vi "Set Speed.vi"(8 "error in (no error)":errorcluster, 10 "speed":dbl, 11 "Masterflex Settings in":T1={"VISA resource name"="", "Simulated?"=FALSE, "Pump Number"=1.0, "Reverse?"=FALSE} {"Pump Number" min=1.0 max=20.0 step=1.0}) -> (0 "error out":errorcluster, 1 "Connection Error":bool, 3 "Masterflex Settings out":T1={"VISA resource name"="", "Simulated?"=FALSE, "Pump Number"=1.0, "Reverse?"=FALSE} {"Pump Number" min=1.0 max=20.0 step=1.0})   [LabVIEW 2018, in "Masterflex 7550-30.lvlib"]
uses:
  Masterflex 7550-30.lvlib
  Controls/Settings Cluster.ctl
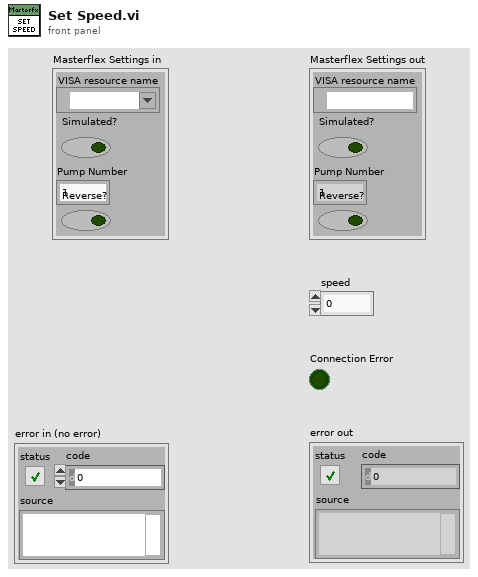
[diagram p1: front panel]
types:
  T1 = typedef "Masterflex 7550-30.lvlib/Settings Cluster.ctl" = cluster{"VISA resource name":refnum<visa-resource-name>, "Simulated?":bool, "Pump Number":dbl, "Reverse?":bool}
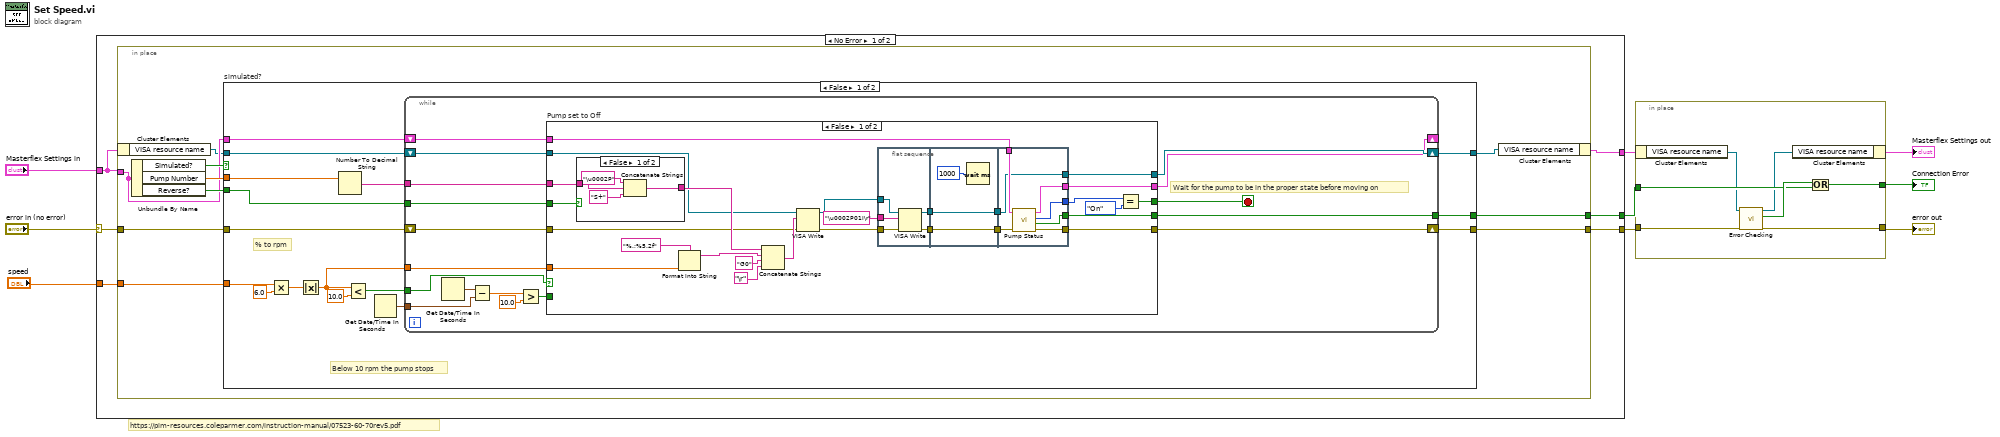
[diagram p0: block diagram]
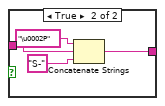
[diagram p2: hidden frame]
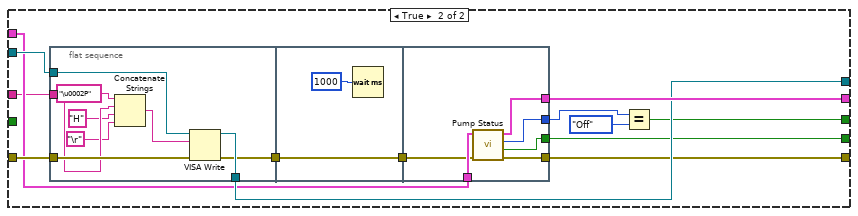
[diagram p3: hidden frame]
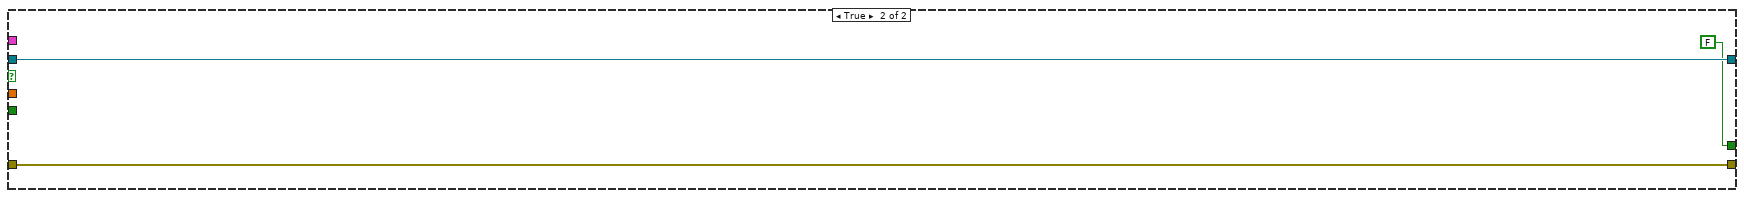
[diagram p4: hidden frame]
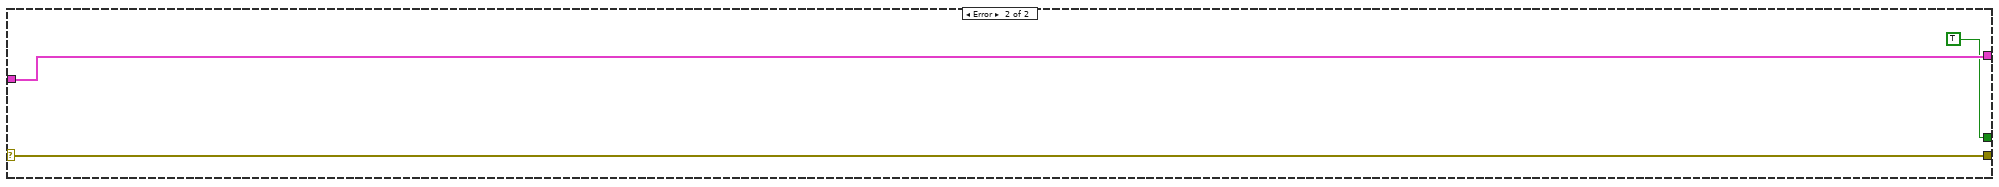
[diagram p5: hidden frame]
diagram:
  # "https://pim-resources.coleparmer.com/instruction-manual/07523-60-70rev5.pdf"
  n1 = case shown="No Error" "error in (no error)" {
    selector: "error in (no error)" -> [w15 w143]
    tunnel: [w14 w143] -> w9
    tunnel: [w10 w142] -> w2
    tunnel: "Masterflex Settings in" -> [w11 w142]
    tunnel: "speed" -> [w13 _]
    tunnel: [w12 TRUE ("Connection Error")] -> w4
    frame No Error {
      n2 = in-place {
        in-place-border: w15 -> [w22]
        in-place-border: [w21] -> w14
        in-place-border: w13 -> [w20]
        in-place-border: w11 -> [w19]
        in-place-border: [w18] -> w12
        n3 = in-place-cluster #1(w11) -> ("VISA resource name"=w17:refnum<visa-resource-name>)
        n4 = Unbundle By Name(w19) -> ("Simulated?"=w24:bool, "Pump Number"=w23:dbl, "Reverse?"=w25:bool)
        n5 = case "simulated?" shown="False" w24 {
          tunnel: w22 -> [w32 w140]
          tunnel: [w39 w140] -> w21
          tunnel: w23 -> [w30 _]
          tunnel: w25 -> [w35 _]
          tunnel: w20 -> [w34 _]
          tunnel: w17 -> [w31 w139]
          tunnel: [w33 w139] -> w16
          tunnel: w19 -> [w27 _]
          tunnel: [w26 FALSE ("Connection Error")] -> w18
          frame False {
            # "% to rpm"
            # "Below 10 rpm the pump stops"
            n6 = Multiply(x=w34, y=6.0) -> (x*y=w37:dbl)
            n7 = Absolute Value(x=w37) -> (abs(x)=w36:dbl)
            n8 = Number To Decimal String(number=w30) -> (decimal integer string=w29:string)  [unwired: 1 in]
            n9 = Less?(x=w36, y=10.0) -> (x < y?=w40:bool)
            n10 = Get Date/Time In Seconds() -> (seconds since 1Jan1904=w28:timestamp)
            n11 = while {
              tunnel: w40 -> [w58]
              tunnel: w36 -> [w56]
              tunnel: w35 -> [w55]
              tunnel: w29 -> [w46]
              shift-right: [w57] -> w39
              shift-left: w32 -> [w48]
              shift-right: [w54] -> w33
              shift-left: w31 -> [w47]
              tunnel: w28 -> [w50]
              shift-right: [w49] -> _
              shift-left: w27 -> [w45]
              tunnel: [w44] -> w26
              stop <- w42 stop-if-true
              # "Wait for the pump to be in the proper state before moving on"
              n12 = Get Date/Time In Seconds() -> (seconds since 1Jan1904=w53:timestamp)
              n13 = Subtract(x=w53, y=w50) -> (x-y=w51:dbl)
              n14 = Greater?(x=w51, y=10.0) -> (0:w43:bool)
              n15 = case "Pump set to Off" shown="False" w58 {
                tunnel: [w70 w114] -> w57
                tunnel: w56 -> [w82 _]
                tunnel: w55 -> [w81 _]
                tunnel: [w71 w116] -> w54
                tunnel: w46 -> [w69 w112]
                tunnel: w43 -> [_ _]
                tunnel: w45 -> [w67 w113]
                tunnel: [w66 w119] -> w49
                tunnel: w48 -> [w64 w120]
                tunnel: w47 -> [w65 w115]
                tunnel: [w63 w111] -> w44
                tunnel: [w59 w108] -> w42
                frame False {
                  n16 = case shown="False" w81 {
                    tunnel: w69 -> [w102 w105]
                    tunnel: [w100 w104] -> w84
                    frame False {
                      n17 = Concatenate Strings("\u0002P" ("string"), w102, "S+" ("string")) -> (w100:string)
                    }
                    frame True {
                      n18 = Concatenate Strings("\u0002P" ("string"), w105, "S-" ("string")) -> (w104:string)
                    }
                  }
                  n19 = Format Into String(format string="%.;%5.2f", w82) -> (resulting string=w83:string)  [unwired: 2 in, 1 out]
                  n20 = Concatenate Strings(w84, w83, "G0" ("string"), "\r") -> (w79:string)
                  n21 = VISA Write(VISA resource name=w65, write buffer=w79, error in (no error)=w64) -> (VISA resource name out=w76:refnum<visa-resource-name>, error out=w78:errorcluster)  [unwired: 1 out]
                  n22 = flat-sequence {
                    tunnel: w78 -> [w89]
                    tunnel: "\u0002P01I\r" ("write buffer") -> [w88]
                    tunnel: w76 -> [w87]
                    tunnel: [w86] -> w75
                    tunnel: [w85] -> w72
                    tunnel: w75 -> [w91]
                    tunnel: [w91] -> w74
                    tunnel: [w90] -> w73
                    tunnel: w72 -> [w90]
                    tunnel: w74 -> [w96]
                    tunnel: w73 -> [w98]
                    tunnel: [w96] -> w71
                    tunnel: [w97] -> w70
                    tunnel: w67 -> [w99]
                    tunnel: [w93] -> w66
                    tunnel: [w95] -> w61
                    tunnel: [w94] -> w63
                    frame #0 {
                      n23 = VISA Write(VISA resource name=w87, write buffer=w88, error in (no error)=w89) -> (VISA resource name out=w86:refnum<visa-resource-name>, error out=w85:errorcluster)  [unwired: 1 out]
                    }
                    frame #1 {
                      n24 = Wait (ms)(milliseconds to wait=u32 1000) -> ()  [unwired: 1 out]
                    }
                    frame #2 {
                      n25 = call "Pump Status.vi"("error in (no error)"=w98, "Masterflex Settings in"=w99) -> ("error out"=w97:errorcluster, "Connection Error"=w94:bool, "Pump On?"=w95:enum16{"Off", "On", "Not Initialized"}, "Masterflex Settings out"=w93:T1)  [unwired: 6 in]
                    }
                  }
                  n26 = Equal?(x=w61, y=enum16{"Off", "On", "Not Initialized"}."On") -> (x = y?=w59:bool)
                }
                frame True {
                  n27 = flat-sequence {
                    tunnel: w120 -> [w128]
                    tunnel: w115 -> [w127]
                    tunnel: w112 -> [w125]
                    tunnel: [w122] -> w116
                    tunnel: [w121] -> w117
                    tunnel: [w130] -> w118
                    tunnel: w117 -> [w130]
                    tunnel: w113 -> [w137]
                    tunnel: [w136] -> w110
                    tunnel: [w135] -> w119
                    tunnel: w118 -> [w134]
                    tunnel: [w133] -> w114
                    tunnel: [w132] -> w111
                    frame #0 {
                      n28 = Concatenate Strings("\u0002P" ("string"), w125, "H" ("string"), "\r") -> (w129:string)
                      n29 = VISA Write(VISA resource name=w127, write buffer=w129, error in (no error)=w128) -> (VISA resource name out=w122:refnum<visa-resource-name>, error out=w121:errorcluster)  [unwired: 1 out]
                    }
                    frame #1 {
                      n30 = Wait (ms)(milliseconds to wait=u32 1000) -> ()  [unwired: 1 out]
                    }
                    frame #2 {
                      n31 = call "Pump Status.vi"("error in (no error)"=w134, "Masterflex Settings in"=w137) -> ("error out"=w133:errorcluster, "Connection Error"=w132:bool, "Pump On?"=w136:enum16{"Off", "On", "Not Initialized"}, "Masterflex Settings out"=w135:T1)  [unwired: 6 in]
                    }
                  }
                  n32 = Equal?(x=w110, y=enum16{"Off", "On", "Not Initialized"}."Off") -> (x = y?=w108:bool)
                }
              }
            }
          }
          frame True {
          }
        }
        n33 = in-place-cluster #1("VISA resource name"=w16) -> (w10:T1)
      }
    }
    frame Error {
    }
  }
  n34 = in-place {
    in-place-border: w9 -> [w150]
    in-place-border: [w149] -> w8
    in-place-border: w4 -> [w147]
    in-place-border: [w146] -> w3
    n35 = in-place-cluster #2(w2) -> ("VISA resource name"=w145:refnum<visa-resource-name>)
    n36 = call "Error Checking.vi"("error in (no error)"=w150, "VISA resource name"=w145) -> ("error out"=w149:errorcluster, "Connection Error"=w148:bool, "VISA resource name"=w144:refnum<visa-resource-name>)  [unwired: 7 in]
    n37 = in-place-cluster #2("VISA resource name"=w144) -> (→"Masterflex Settings out":T1)
    n38 = Or(x=w148, y=w147) -> (x .or. y?=w146:bool)
  }
  "error out" <- w8
  "Connection Error" <- w3
